vi "Transcation.vi"(8 "error in (no error)":errorcluster, 10 "Action":enum16{"begin", "commit", "rollback"}(ring), 11 "ODBC-Interface in":refnum<class "ODBC-Interface.lvclass">) -> (0 "error out":errorcluster, 3 "ODBC-Interface out":refnum<class "ODBC-Interface.lvclass">)   [LabVIEW 2012, in "DB-Configuration.lvlib" / "ODBC-Interface.lvclass"]
doc: "Begin, commit or rollback a transaction."
uses:
  ODBC-Interface.lvclass
  ODBC-Interface.lvclass/ODBC-Interface.ctl
  <vilib>/addons/database/Connection.llb/Conn Transaction.vi
  <vilib>/addons/database/NI_Database_API.lvlib
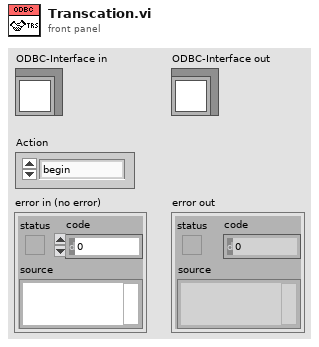
[diagram p1: front panel]
types:
  T1 = typedef "NI_Database_API.lvlib/Conn ObjectReference.ctl" = refnum<k1>
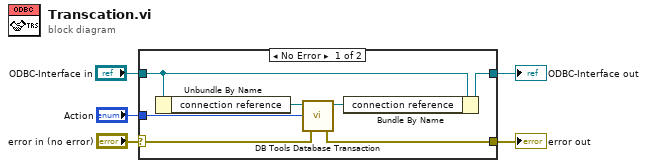
[diagram p0: block diagram]
diagram:
  n1 = case shown="No Error" "error in (no error)" {
    selector: "error in (no error)" -> [w6 w13]
    tunnel: "Action" -> [w12 _]
    tunnel: "ODBC-Interface in" -> [w10 w14]
    tunnel: [w8 w13] -> w3
    tunnel: [w7 w14] -> w2
    frame No Error {
      n2 = Unbundle By Name(w10) -> ("connection reference"=w11:T1)
      n3 = call-poly <vilib>:"DB Tools Database Transaction.vi"("error in (no error)"=w6, "operation (begin)"=w12, "connection reference"=w11) -> ("error out"=w8:errorcluster, "connection reference out"=w9:T1)  [unwired: 3 in]
      n4 = Bundle By Name(cluster=w10, "connection reference"=w9) -> (w7:refnum<class "ODBC-Interface.lvclass">)
    }
    frame Error {
    }
  }
  "error out" <- w3
  "ODBC-Interface out" <- w2
